vi "SubVI_Cluster_Array.vi"(8 "Z Array in":dbl[](array[numeric]), 9 "Y Array in":dbl[](array[numeric]), 10 "X Array in":dbl[](array[numeric]), 11 "Angular Displacement Feedback (Gyro)":dbl[](array[numeric])) -> (0 "Appended array":dbl[][](array[numeric]), 1 "Z Out":dbl[](array[numeric]), 2 "Y Out":dbl[](array[numeric]), 3 "X Out":dbl[](array[numeric]))   [LabVIEW 2014]
uses:
  Globals_Real.vi
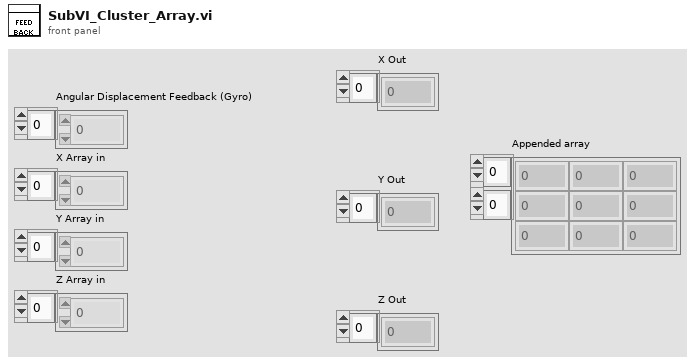
[diagram p1: front panel]
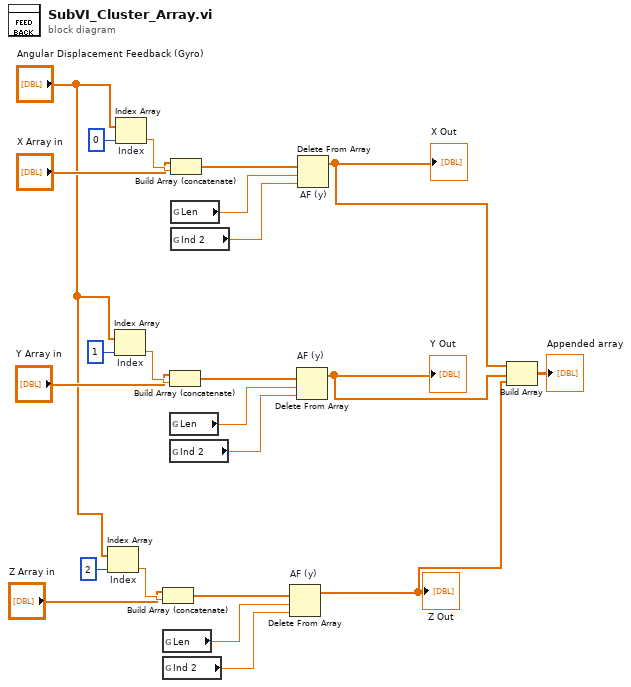
[diagram p0: block diagram]
diagram:
  n1 = Index Array "Index"(array="Angular Displacement Feedback (Gyro)", index=2) -> (element=w10:dbl)
  n2 = Index Array "Index"(array="Angular Displacement Feedback (Gyro)", index=1) -> (element=w16:dbl)
  n3 = Index Array "Index"(array="Angular Displacement Feedback (Gyro)", index=0) -> (element=w22:dbl)
  n4 = Build Array (concatenate) "Build Array"("Z Array in", w10) -> (w11:dbl[])
  n5 = global read "Globals_Real.vi" "Len"() -> (w6:dbl)
  n6 = global read "Globals_Real.vi" "Ind 2"() -> (w7:dbl)
  n7 = Build Array (concatenate) "Build Array"("Y Array in", w16) -> (w17:dbl[])
  n8 = global read "Globals_Real.vi" "Len"() -> (w12:dbl)
  n9 = global read "Globals_Real.vi" "Ind 2"() -> (w13:dbl)
  n10 = Build Array (concatenate) "Build Array"("X Array in", w22) -> (w23:dbl[])
  n11 = global read "Globals_Real.vi" "Len"() -> (w18:dbl)
  n12 = global read "Globals_Real.vi" "Ind 2"() -> (w19:dbl)
  n13 = Delete From Array "AF (y)"(array=w11, length=w6, index=w7) -> (array with subset deleted=w2:dbl[])  [unwired: 1 out]
  "Z Out" <- w2
  n14 = Delete From Array "AF (y)"(array=w17, length=w12, index=w13) -> (array with subset deleted=w3:dbl[])  [unwired: 1 out]
  "Y Out" <- w3
  n15 = Delete From Array "AF (y)"(array=w23, length=w18, index=w19) -> (array with subset deleted=w4:dbl[])  [unwired: 1 out]
  "X Out" <- w4
  n16 = Build Array(w4, w3, w2) -> (→"Appended array":dbl[][])
